vi "database_no_data.vi"(3 "input":string) -> (1 "error":errorcluster)   [LabVIEW 2017, in "Lib_code.lvlib"]
uses:
  Lib_code.lvlib
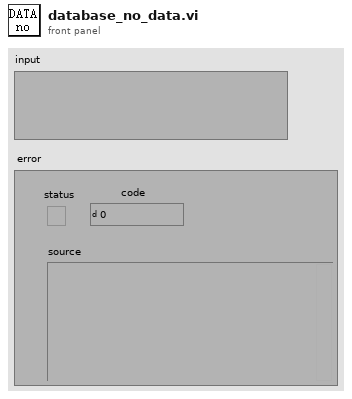
[diagram p1: front panel]
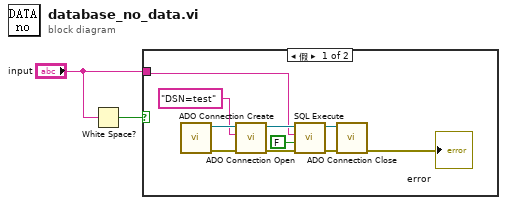
[diagram p0: block diagram]
diagram:
  n1 = White Space?(1:"input") -> (0:w2:bool)
  n2 = case shown="假" w2 {
    tunnel: "input" -> [w3 _]
    frame False {
      n3 = call <userlib>:"ADO Connection Create.vi"() -> ("error out"=w9:errorcluster, "ADODB._Connection Out"=w6:refnum<k7>)  [unwired: 10 in]
      n4 = call <userlib>:"ADO Connection Open.vi"("error in (no error)"=w9, "ConnectionString"="DSN=test", "ADODB._Connection In"=w6) -> ("error out"=w10:errorcluster, "ADODB._Connection Out"=w7:refnum<k7>)  [unwired: 7 in]
      n5 = call <userlib>:"SQL Execute.vi"("error in (no error)"=w10, "Return Data (T)"=FALSE, "Command Text"=w3, "ADODB._Connection In"=w7) -> ("error out"=w11:errorcluster, "ADODB._Connection Out"=w8:refnum<k7>)  [unwired: 4 in, 2 out]
      n6 = call <userlib>:"ADO Connection Close.vi"("error in (no error)"=w11, "ADODB._Connection In"=w8) -> ("error out"=→"error":errorcluster)  [unwired: 8 in, 1 out]
    }
    frame True {
    }
  }
